vi "q4 simple interest.vi"(9 "T":dbl, 10 "R":dbl, 11 "P":dbl) -> (1 "SI":dbl)   [LabVIEW 2025]
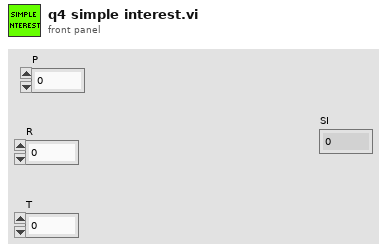
[diagram p1: front panel]
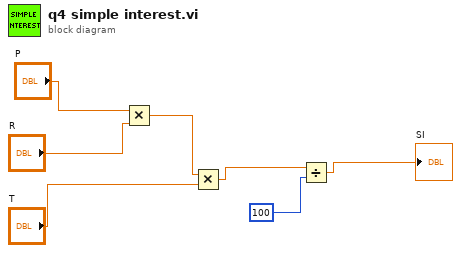
[diagram p0: block diagram]
diagram:
  n1 = Multiply(x="P", y="R") -> (x*y=w5:dbl)
  n2 = Multiply(x=w5, y="T") -> (x*y=w3:dbl)
  n3 = Divide(x=w3, y=100) -> (x/y=→"SI":dbl)
